vi "TRIGger.vi"(4 "Timeout (ms)":u32=1000, 5 "Continuous":bool, 6 "Period (s)":dbl=0.1 min=0.000488 max=2.79 format="%^#_3g", 7 "Count":u16=1 min=1 max=4096 step=1, 8 "Error in (no error)":errorcluster, 9 "Source":enum16{"IMMediate", "TIMer", "BUS"}(ring), 10 "Function":T1(ring)=enum."Setup query", 11 "VISA resource":refnum<visa-resource-name>) -> (0 "Error out":errorcluster, 2 "Response":string, 3 "Dup VISA resource":refnum<visa-resource-name>)   [LabVIEW 2010]
doc: "Copyright (c) 2012 Metrolab Technology SA, Plan-les-Ouates, Geneva, Switzerland\nManages all functions of trigger system."
panel:
  # "TRIGger"
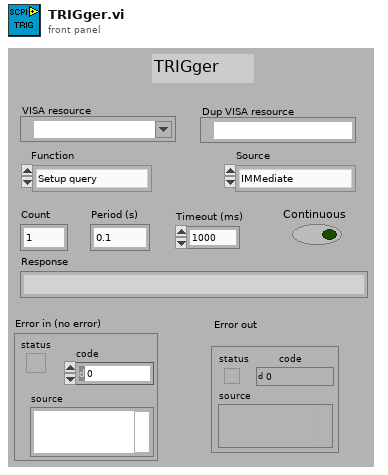
[diagram p1: front panel]
types:
  T1 = enum16{"Setup", "Setup query", "INITiate", "ABORt"}
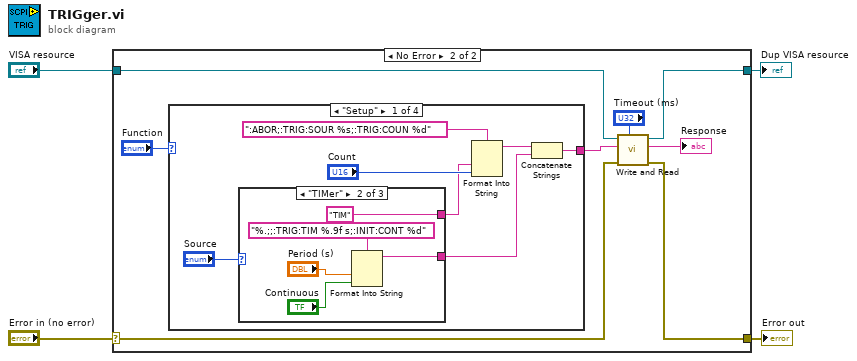
[diagram p0: block diagram]
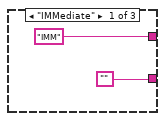
[diagram p3: hidden frame]
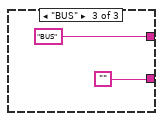
[diagram p4: hidden frame]
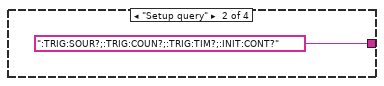
[diagram p5: hidden frame]
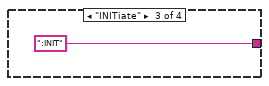
[diagram p6: hidden frame]
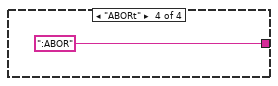
[diagram p7: hidden frame]
diagram:
  n1 = case shown="No Error" "Error in (no error)" {
    selector: "Error in (no error)" -> [w5 w11]
    tunnel: "VISA resource" -> [w6 w14]
    tunnel: [w6 w10] -> w1
    tunnel: [w5 w9] -> w4
    frame Error {
    }
    frame No Error {
      n2 = case shown="\"Setup\"" "Function" {
        tunnel: [w17 ":TRIG:SOUR?;:TRIG:COUN?;:TRIG:TIM?;:INIT:CONT?" ("format string") ":INIT" ("format string") ":ABOR" ("format string")] -> w8
        frame "Setup" {
          n3 = case shown="\"TIMer\"" "Source" {
            tunnel: ["" w25 ""] -> w16
            tunnel: ["IMM" ("format string") "TIM" ("format string") "BUS" ("format string")] -> w15
            frame "IMMediate" {
            }
            frame "TIMer" {
              n4 = Format Into String(format string="%.;;:TRIG:TIM %.9f s;:INIT:CONT %d", "Period (s)", "Continuous") -> (resulting string=w25:string)  [unwired: 2 in, 1 out]
            }
            frame "BUS" {
            }
          }
          n5 = Format Into String(format string=":ABOR;:TRIG:SOUR %s;:TRIG:COUN %d", w15, "Count") -> (resulting string=w19:string)  [unwired: 2 in, 1 out]
          n6 = Concatenate Strings(w19, w16) -> (w17:string)
        }
        frame "Setup query" {
        }
        frame "INITiate" {
        }
        frame "ABORt" {
        }
      }
      n7 = call "Write and Read.vi"("Timeout (ms)"="Timeout (ms)", "Error in (no error)"=w11, "Command"=w8, "VISA resource"=w14) -> ("Error out"=w9:errorcluster, "Response"=→"Response":string, "Dup VISA resource"=w10:refnum<visa-resource-name>)  [unwired: 3 in, 2 out]
    }
  }
  "Error out" <- w4
  "Dup VISA resource" <- w1
